vi "Mercury_GoToField.vi"(8 "error in":errorcluster, 10 "persistent mode":bool=TRUE, 11 "Mercury Targets":T1={"Target Field (T)"=0.1, "Target Field Rate (T/min)"=0.1} {"Target Field (T)" format="%.4g"; "Target Field Rate (T/min)" format="%.4g"}) -> (0 "error out":errorcluster)   [LabVIEW 2016]
doc: "Use this VI to remotely interact with the Oxford Mercury power supply through \"Oxford-1820-Main.vi\", which MUST also be running."
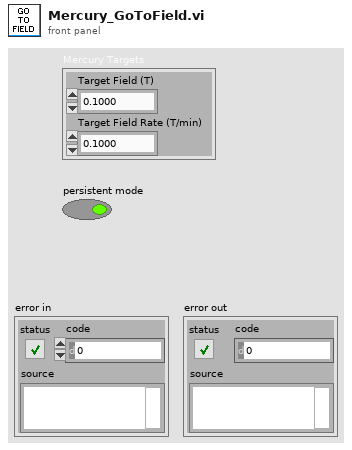
[diagram p1: front panel]
types:
  T1 = cluster{"Target Field (T)":dbl, "Target Field Rate (T/min)":dbl}
  T2 = cluster{"Magnet Field":dbl, "PS Field":dbl, "Target Field":dbl, "Target Field Rate":dbl, "Voltage":dbl, "Current":dbl, "Switch":bool}
  T3 = cluster{"Hold":bool, "Clamp":bool, "To Set":bool, "To Zero":bool, "Send to IPS":bool, "PS Heat":bool, "Lambda":bool}
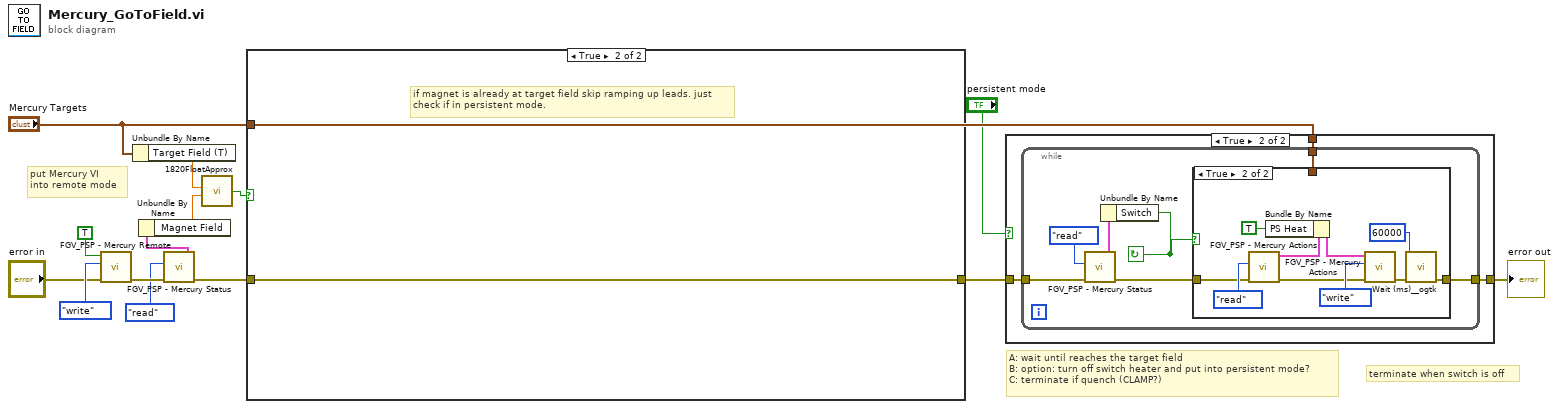
[diagram p0: block diagram]
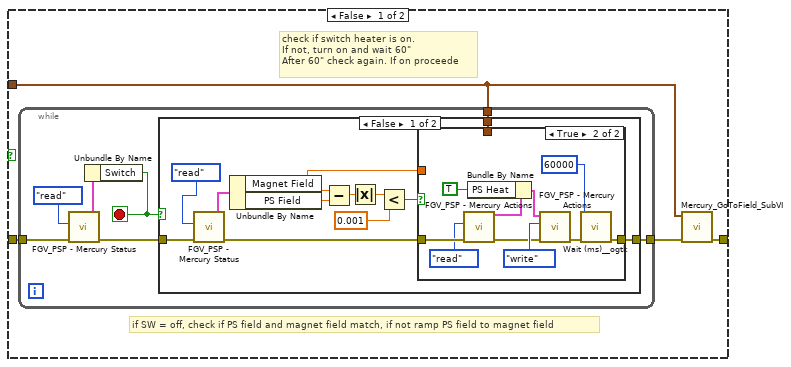
[diagram p2: hidden frame]
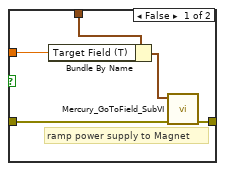
[diagram p3: hidden frame]
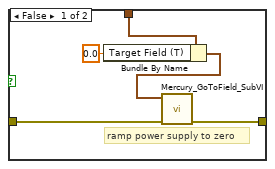
[diagram p6: hidden frame]
diagram:
  # "terminate when switch is off"
  # "A: wait until reaches the target field\nB: option: turn off switch heater and put into persistent mode?\nC: terminate if quench (CLAMP?)"
  # "put Mercury VI\ninto remote mode"
  n1 = call "FGV_PSP - Mercury Remote.vi"("error in"="error in", "Function"=enum16{"write", "read"}."write", "Mercury Remote"=TRUE) -> ("error out"=w12:errorcluster)  [unwired: 3 in, 1 out]
  n2 = Unbundle By Name("Mercury Targets") -> ("Target Field (T)"=w6:dbl)
  n3 = call "FGV_PSP - Mercury Status.vi"("error in"=w12, "Function"=enum16{"write", "read"}."read") -> ("error out"=w11:errorcluster, "status"=w10:T2)  [unwired: 4 in]
  n4 = Unbundle By Name(w10) -> ("Magnet Field"=w3:dbl)
  n5 = call "1820FloatApprox.vi"("y"=w3, "x"=w6) -> ("x ~ y?"=w5:bool)  [unwired: 2 in]
  n6 = case shown="True" w5 {
    tunnel: w11 -> [w18 w54]
    tunnel: [w16 w54] -> w9
    tunnel: "Mercury Targets" -> [w15 _]
    frame False {
      # "if SW = off, check if PS field and magnet field match, if not ramp PS field to magnet field"
      # "check if switch heater is on.\nIf not, turn on and wait 60\"\nAfter 60\" check again. If on proceede"
      n7 = while {
        tunnel: [w22] -> w17
        tunnel: w18 -> [w21]
        tunnel: w15 -> [w19]
        stop <- w23 stop-if-true
        n8 = call "FGV_PSP - Mercury Status.vi"("error in"=w21, "Function"=enum16{"write", "read"}."read") -> ("error out"=w24:errorcluster, "status"=w25:T2)  [unwired: 4 in]
        n9 = Unbundle By Name(w25) -> ("Switch"=w23:bool)
        n10 = case shown="False" w23 {
          tunnel: w24 -> [w36 w53]
          tunnel: [w37 w53] -> w22
          tunnel: w19 -> [w28 _]
          frame False {
            n11 = call "FGV_PSP - Mercury Status.vi"("error in"=w36, "Function"=enum16{"write", "read"}."read") -> ("error out"=w34:errorcluster, "status"=w35:T2)  [unwired: 4 in]
            n12 = Unbundle By Name(w35) -> ("Magnet Field"=w27:dbl, "PS Field"=w33:dbl)
            n13 = Subtract(x=w27, y=w33) -> (x-y=w32:dbl)
            n14 = Absolute Value(x=w32) -> (abs(x)=w31:dbl)
            n15 = Less?(x=w31, y=0.001) -> (x < y?=w29:bool)
            n16 = case shown="True" w29 {
              tunnel: [w41 w49] -> w37
              tunnel: w34 -> [w42 w47]
              tunnel: w28 -> [w40 _]
              tunnel: w27 -> [w39 _]
              frame False {
                # "ramp power supply to Magnet"
                n17 = Bundle By Name(cluster=w40, "Target Field (T)"=w39) -> (w38:T1)
                n18 = call "Mercury_GoToField_SubVI.vi"("error in (no error)"=w42, "Mercury Targets"=w38) -> ("error out"=w41:errorcluster)  [unwired: 9 in]
              }
              frame True {
                n19 = call "FGV_PSP - Mercury Actions.vi"("error in"=w47, "Function"=enum16{"write", "read"}."read") -> ("error out"=w46:errorcluster, "mercury actions 2"=w44:T3)  [unwired: 4 in]
                n20 = Bundle By Name(cluster=w44, "PS Heat"=TRUE ("Send to IPS")) -> (w43:T3)
                n21 = call "FGV_PSP - Mercury Actions.vi"("error in"=w46, "Function"=enum16{"write", "read"}."write", "mercury actions"=w43) -> ("error out"=w50:errorcluster)  [unwired: 3 in, 1 out]
                n22 = call <userlib>:"Wait (ms)__ogtk.vi"("error in (no error)"=w50, "milliseconds to wait"=u32 60000) -> ("error out"=w49:errorcluster)  [unwired: 8 in, 1 out]
              }
            }
          }
          frame True {
          }
        }
      }
      n23 = call "Mercury_GoToField_SubVI.vi"("error in (no error)"=w17, "Mercury Targets"=w15) -> ("error out"=w16:errorcluster)  [unwired: 9 in]
    }
    frame True {
      # "if magnet is already at target field skip ramping up leads. just\ncheck if in persistent mode."
    }
  }
  n24 = case shown="True" "persistent mode" {
    tunnel: w9 -> [w55 w58]
    tunnel: "Mercury Targets" -> [_ w57]
    tunnel: [w55 w56] -> w8
    frame False {
    }
    frame True {
      n25 = while {
        tunnel: [w64] -> w56
        tunnel: w58 -> [w59]
        tunnel: w57 -> [w62]
        stop <- w61 continue-if-true
        n26 = call "FGV_PSP - Mercury Status.vi"("error in"=w59, "Function"=enum16{"write", "read"}."read") -> ("error out"=w60:errorcluster, "status"=w65:T2)  [unwired: 4 in]
        n27 = Unbundle By Name(w65) -> ("Switch"=w61:bool)
        n28 = case shown="True" w61 {
          tunnel: [w70 w77] -> w64
          tunnel: w62 -> [w69 _]
          tunnel: w60 -> [w66 w71]
          frame False {
            # "ramp power supply to zero"
            n29 = Bundle By Name(cluster=w69, "Target Field (T)"=0.0) -> (w68:T1)
            n30 = call "Mercury_GoToField_SubVI.vi"("error in (no error)"=w66, "Mercury Targets"=w68) -> ("error out"=w70:errorcluster)  [unwired: 9 in]
          }
          frame True {
            n31 = call "FGV_PSP - Mercury Actions.vi"("error in"=w71, "Function"=enum16{"write", "read"}."read") -> ("error out"=w75:errorcluster, "mercury actions 2"=w74:T3)  [unwired: 4 in]
            n32 = Bundle By Name(cluster=w74, "PS Heat"=TRUE ("Send to IPS")) -> (w73:T3)
            n33 = call "FGV_PSP - Mercury Actions.vi"("error in"=w75, "Function"=enum16{"write", "read"}."write", "mercury actions"=w73) -> ("error out"=w78:errorcluster)  [unwired: 3 in, 1 out]
            n34 = call <userlib>:"Wait (ms)__ogtk.vi"("error in (no error)"=w78, "milliseconds to wait"=u32 60000) -> ("error out"=w77:errorcluster)  [unwired: 8 in, 1 out]
          }
        }
      }
    }
  }
  "error out" <- w8
